vi "maps.vi"() -> ()   [LabVIEW 2015]
panel:
  in  "stop":bool
  in  "Zoom":i32(slide) scale=1.0..20.0
  in  "Long":dbl
  in  "Lat":dbl
  in  "WebBrowser":refnum<k7>(container)
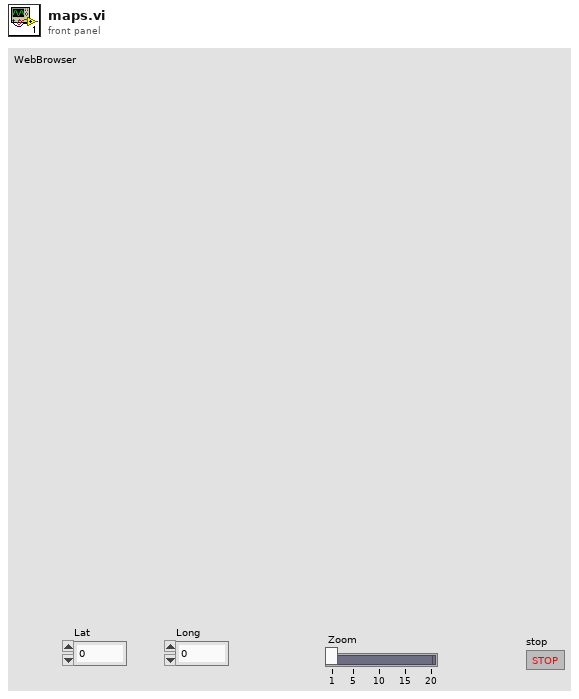
[diagram p1: front panel]
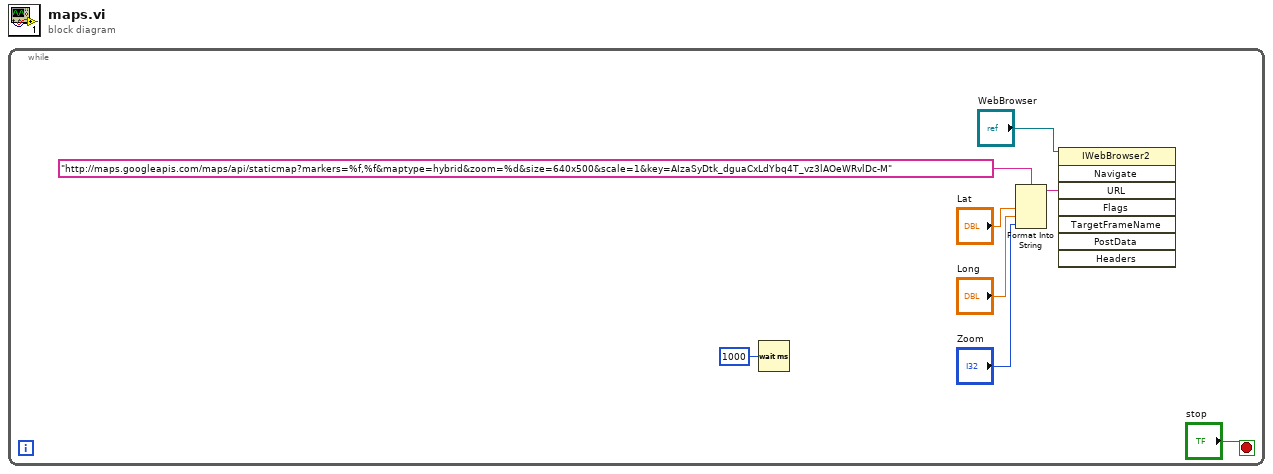
[diagram p0: block diagram]
diagram:
  n1 = while {
    stop <- "stop" stop-if-true
    n2 = Wait (ms)(milliseconds to wait=u32 1000) -> ()  [unwired: 1 out]
    n3 = Format Into String(format string="http://maps.googleapis.com/maps/api/staticmap?markers=%f,%f&maptype=hybrid&zoom=%d&size=640x500&scale=1&key=AIzaSyDtk_dguaCxLdYbq4T_vz3lAOeWRvlDc-M", "Lat", "Long", "Zoom") -> (resulting string=w3:string)  [unwired: 2 in, 1 out]
    n4 = invoke class="IWebBrowser2" method="Navigate"(reference="WebBrowser", "URL"=w3) -> ()  [unwired: 6 in, 8 out]
  }
